vi "Write Image Header.vi"(8 "error in (no error)":errorcluster, 11 "CCDCamera in":refnum<class "CCDCamera.lvclass">) -> (0 "error out":errorcluster, 3 "CCDCamera out":refnum<class "CCDCamera.lvclass">)   [LabVIEW 2018, in "CCDCamera.lvclass"]
uses:
  CCDCamera.lvclass
  <userlib>/gfitsio/gfitsio.lvlib
  <userlib>/gfitsio/gfitsio-write-key-string.vi
panel:
  in  "Header Contents":T1={"FILENAME"=["FILENAME", "example.fits", "File name at acquisition"], "OBSERVER"=["OBSERVER", "Denis", "Name of the observer"], "PROGRID"=["PROGRID", "2018A-001", "Program ID"], "OBJECT"=["OBJECT", "UNDEFINED", "Object name"], "NIGHTDIR"=["NIGHTDIR", "DIR", "Night directory name "], "CHANNEL"=["CHANNEL", "RED", "Instrument channel"], "INSTRUME"=["INSTRUME", "ECHARPE", "Instrument"], "NEXPSEQ"=["NEXPSEQ", "1", "Total number of exposures in sequence"], "SEQINDEX"=["SEQINDEX", "1", "Exposure index in the sequence"], "OBSTYPE"=["OBSTYPE", "BIAS", "Image type: OBJECT, BIAS, FLAT, ARC, DARK"], "READOUT"=["READOUT", "Normal", "Read out rate"], "SHUTTER"=["SHUTTER", "CLOSED", "Shutter Mode (OPEN, CLOSED, or AUTO) "], "OPENSHT"=["OPENSHT", "50", "Time to open the shutter (ms) "], "CLOSESHT"=["CLOSESHT", "50", "Time to close the shutter (ms)"], "EM GAIN"=["EMGAIN", "2", "Electron Multiplying gain"], "EMMODE "=["EMMODE", "Electron Multiplying", "Electron Multiplying Mode"], "EXPTIME"=["EXPTIME", "1", "Exposure time (s)"], "PREAMP GAIN"=["PREAMP", "3.38", "Pre-amplifier gain"], "VSHIFT"=["VSHIFT", "4.33", "Vertical Shift Spedd (usec)"], "ACQMODE"=["ACQMODE", "SINGLE", "Acquisition Mode"], "TRIGGER"=["TRIGGER", "internal", "Trigger Mode"], "READMODE"=["READMODE", "Single", "Read Mode"], "SHUTTTL"=["SHUTTTL", "TTL LOW", "Shutter TTL"], "HBIN"=["HBIN", "1", "Horizontal Binning"], "INITLINE"=["INITLINE", "1", "Initial Line Multiplying gain"], "INITCOL"=["INITCOL", "1 ", "Initial Column"], "FINALLIN"=["FINALLIN", "1024", "Final Line"], "VBIN"=["VBIN", "1", "Vertical Binning"], "FINALCOL"=["FINALCOL", "1024", "Final Column"]}
  out "Camera Setup":T2={"Image Name"="Image", "Image Path"="C:\\Users\\Cliente\\Desktop\\SPARC4_AC\\Imagens\\", "# Images"="", "Exposure Time"="", "Pre-amp gain"="", "Readout Rate"="", "Vertical Shift Speed"="", "Acquisition Mode"="", "Trigger"="", "Read Mode"="", "EM Mode"="", "EM Gain"="", "Shutter Mode"="", "Shutter TTL"="", "Time to open shutter"="", "Time to close shutter"="", "Vertical Binning"="", "Horizontal Binning"="", "Initial Line"="", "Initial Cloumn"="", "Final Line"="", "Final Column"="", "#img in sequence"=""}
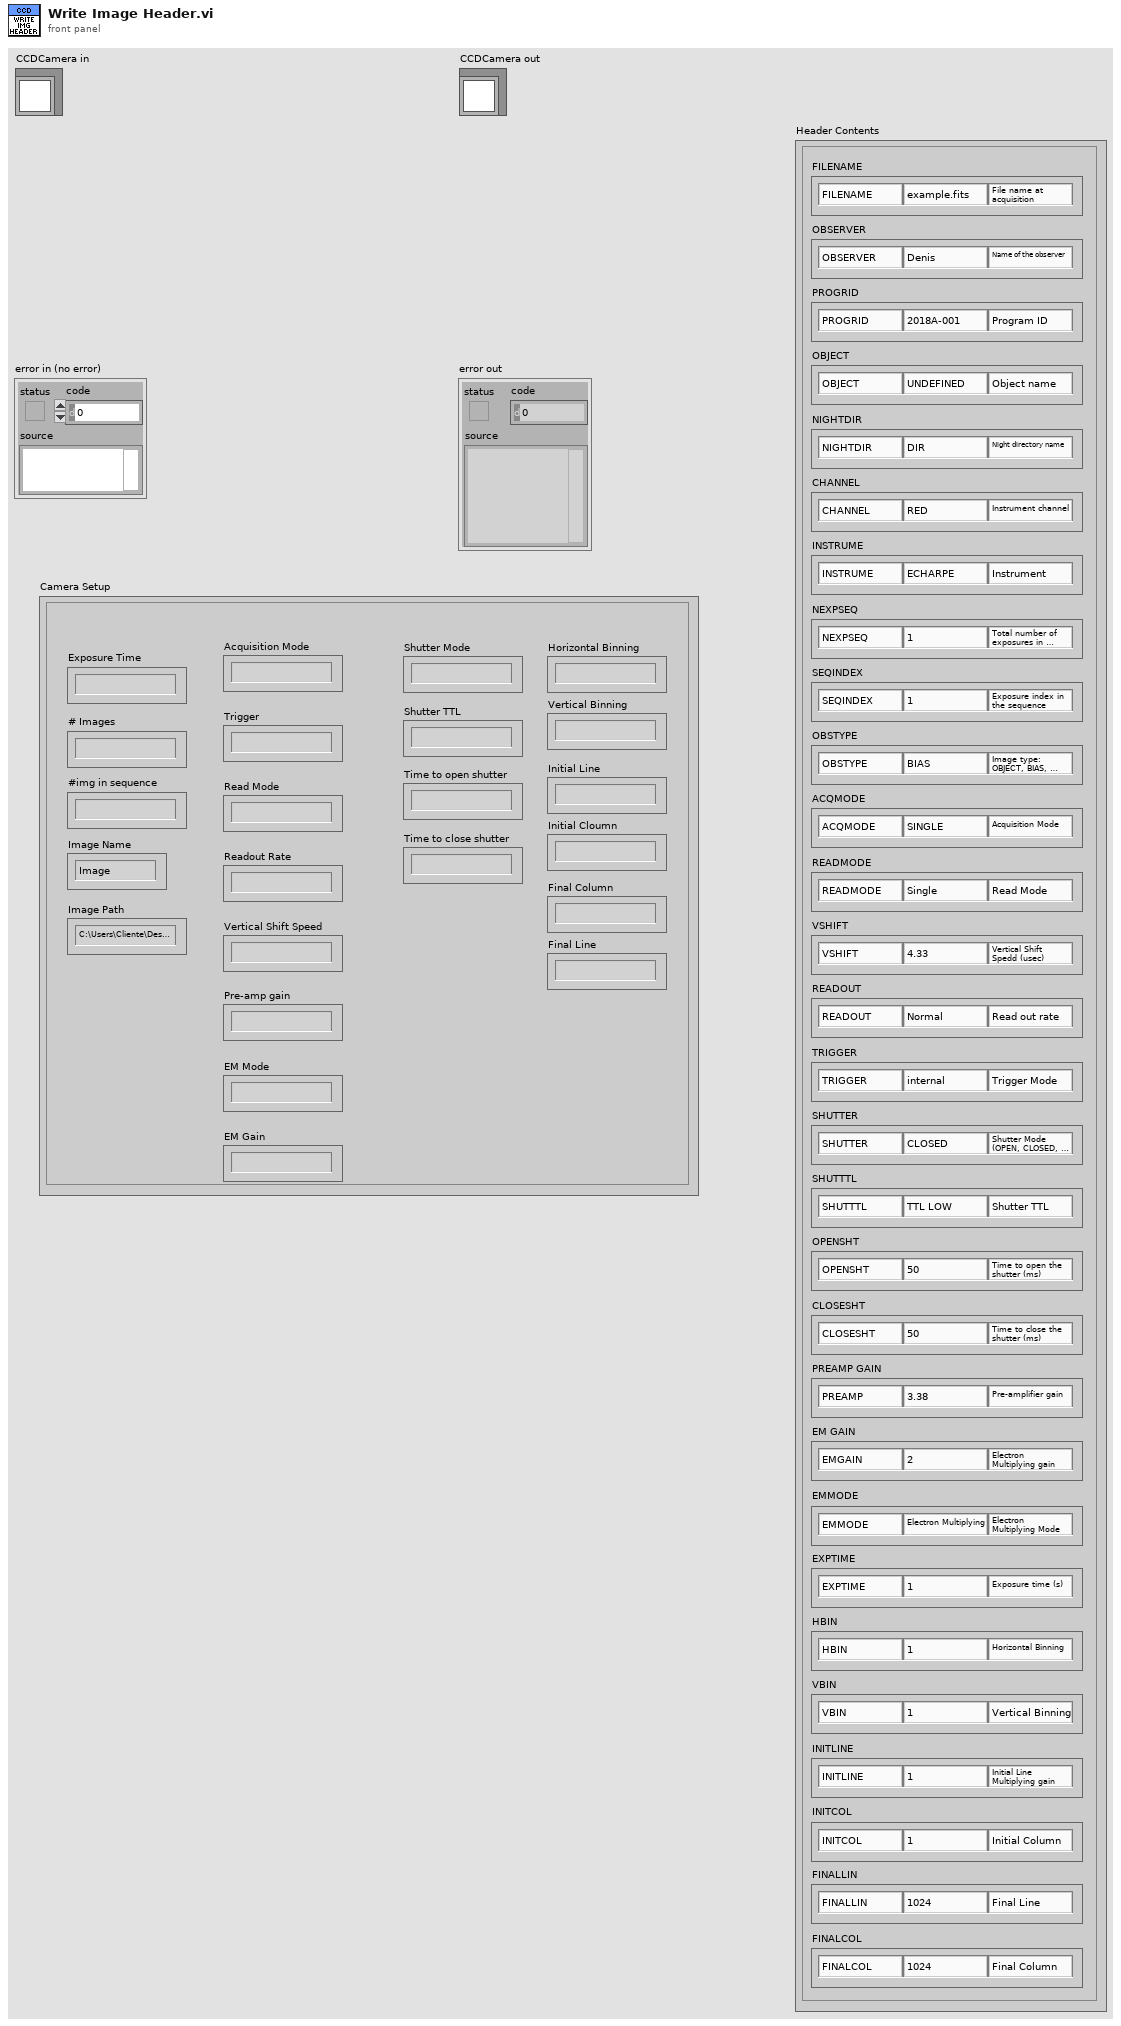
[diagram p1: front panel]
types:
  T1 = cluster{"FILENAME":string[], "OBSERVER":string[], "PROGRID":string[], "OBJECT":string[], "NIGHTDIR":string[], "CHANNEL":string[], "INSTRUME":string[], "NEXPSEQ":string[], "SEQINDEX":string[], "OBSTYPE":string[], "READOUT":string[], "SHUTTER":string[], "OPENSHT":string[], "CLOSESHT":string[], "EM GAIN":string[], "EMMODE ":string[], "EXPTIME":string[], "PREAMP GAIN":string[], "VSHIFT":string[], "ACQMODE":string[], "TRIGGER":string[], "READMODE":string[], "SHUTTTL":string[], "HBIN":string[], "INITLINE":string[], "INITCOL":string[], "FINALLIN":string[], "VBIN":string[], "FINALCOL":string[]}
  T2 = cluster{"Image Name":string, "Image Path":string, "# Images":string, "Exposure Time":string, "Pre-amp gain":string, "Readout Rate":string, "Vertical Shift Speed":string, "Acquisition Mode":string, "Trigger":string, "Read Mode":string, "EM Mode":string, "EM Gain":string, "Shutter Mode":string, "Shutter TTL":string, "Time to open shutter":string, "Time to close shutter":string, "Vertical Binning":string, "Horizontal Binning":string, "Initial Line":string, "Initial Cloumn":string, "Final Line":string, "Final Column":string, "#img in sequence":string}
  T3 = cluster{"Image Name":string, "Image Path":string, "# Images":u32, "Exposure Time":dbl, "Pre-amp gain":u8, "Readout Rate":u8, "Vertical Shift Speed":u8, "Acquisition Mode":u8, "Trigger":u8, "Read Mode":u8, "EM Mode":u8, "EM Gain":u16, "Shutter Mode":u8, "Shutter TTL":u8, "Time to open shutter":u16, "Time to close shutter":u16, "Vertical Binning":u16, "Horizontal Binning":u16, "Initial Line":u16, "Initial Column":u16, "Final Line":u16, "Final Column":u16, "Image Name (TEMP)":string, "#img in sequence":u32, "Kinetic Series Length":u32, "Number of Accumulations":u32, "Kinetic Cycle Time":u32, "Frame Transfer":bool, "Vertical Clock Amplitude":u8}
  T4 = enum16{"open", "open or create", "create or replace", "create", "open (read only)"}
  T5 = typedef "gfitsio.lvlib/gfitsio-refnum.ctl" = refnum<k1>
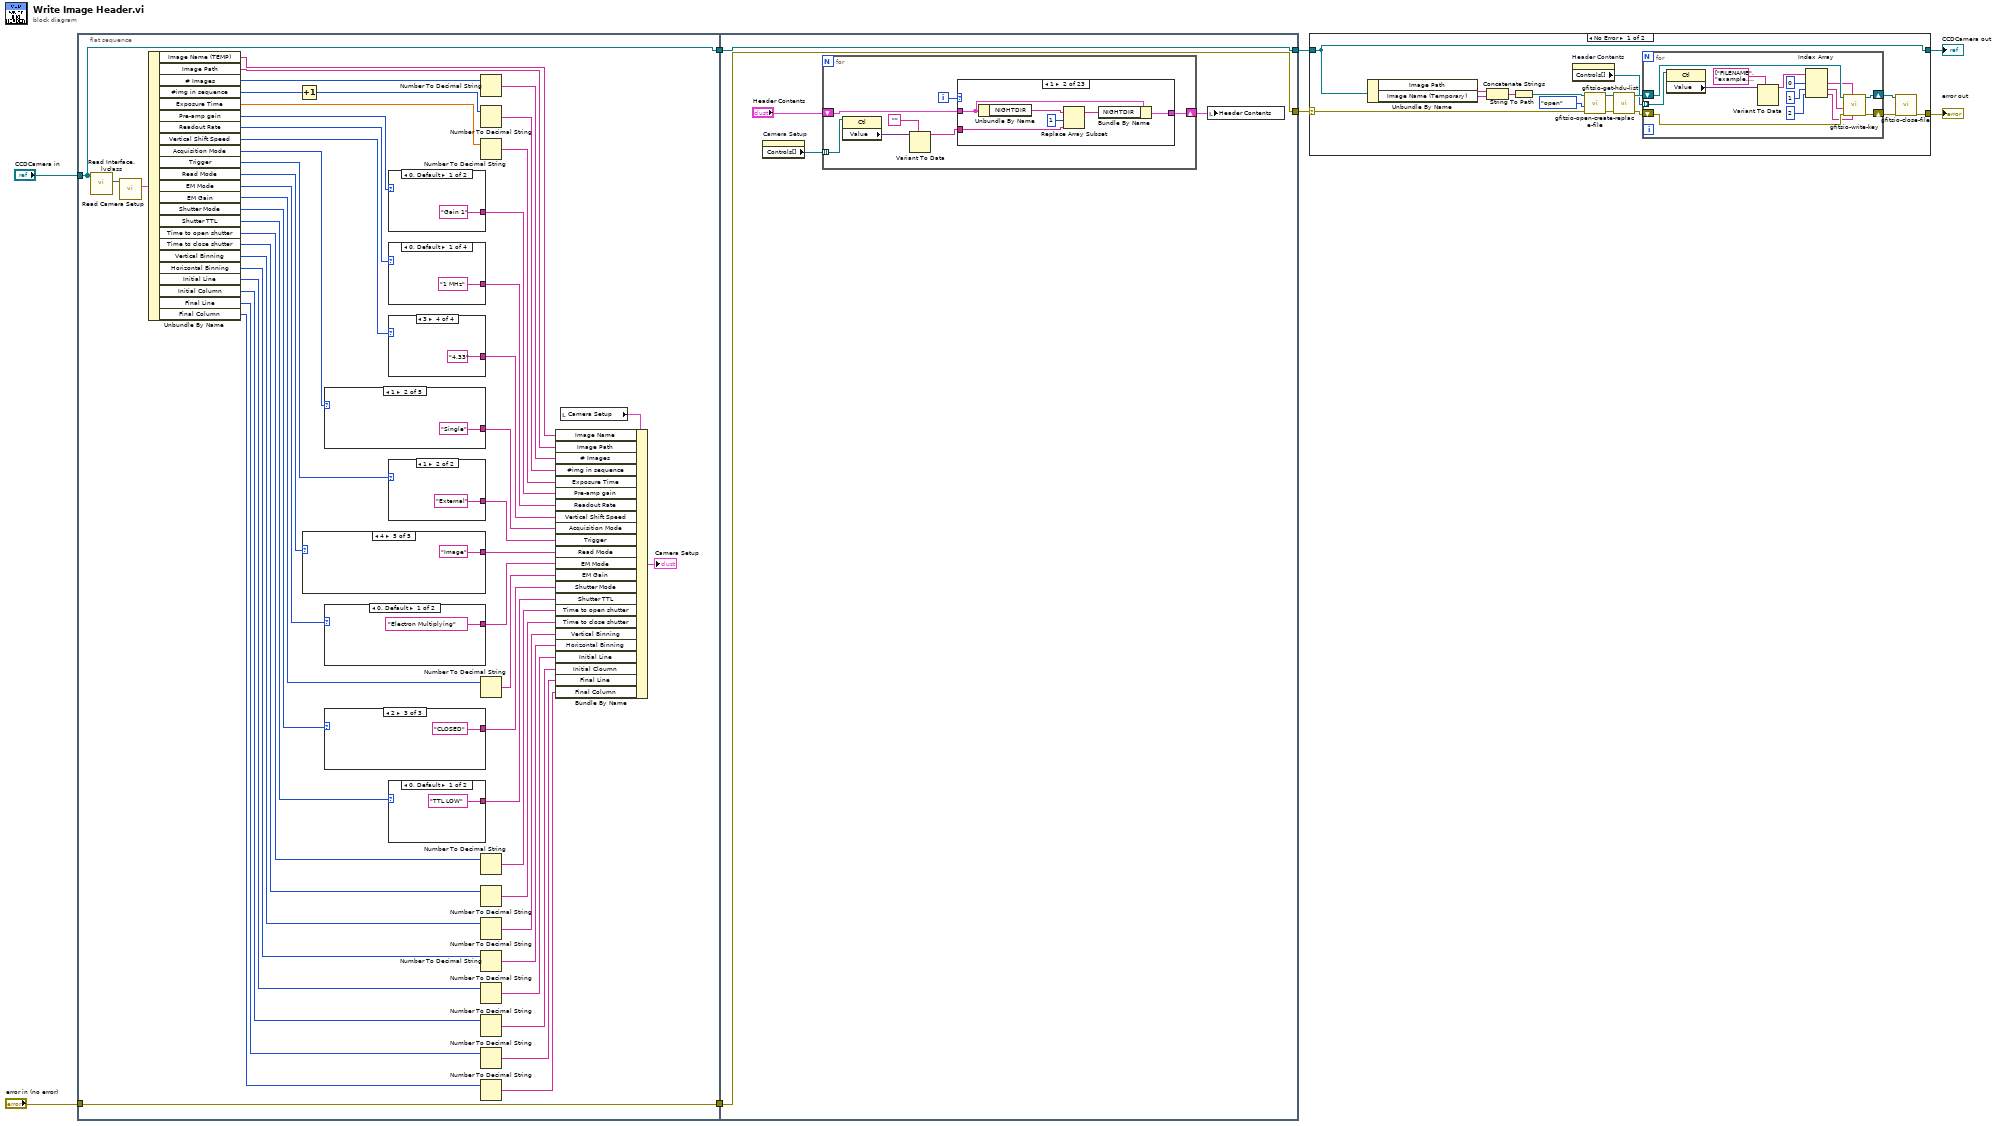
[diagram p0: block diagram]
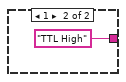
[diagram p2: hidden frame]
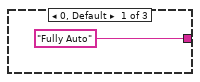
[diagram p3: hidden frame]
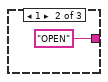
[diagram p4: hidden frame]
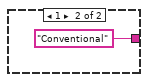
[diagram p5: hidden frame]
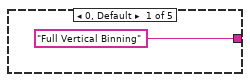
[diagram p6: hidden frame]
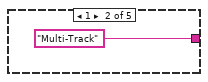
[diagram p7: hidden frame]
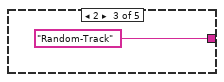
[diagram p8: hidden frame]
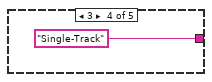
[diagram p9: hidden frame]
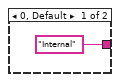
[diagram p10: hidden frame]
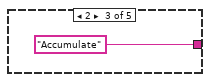
[diagram p12: hidden frame]
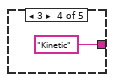
[diagram p13: hidden frame]
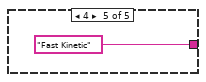
[diagram p14: hidden frame]
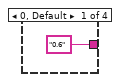
[diagram p15: hidden frame]
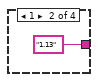
[diagram p16: hidden frame]
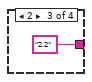
[diagram p17: hidden frame]
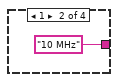
[diagram p18: hidden frame]
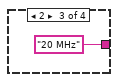
[diagram p19: hidden frame]
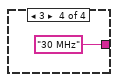
[diagram p20: hidden frame]
diagram:
  n1 = flat-sequence {
    tunnel: "CCDCamera in" -> [w13]
    tunnel: [w13] -> w5
    tunnel: [w12] -> w4
    tunnel: "error in (no error)" -> [w12]
    tunnel: w5 -> [w90]
    tunnel: w4 -> [w89]
    tunnel: [w90] -> w2
    tunnel: [w89] -> w1
    frame #0 {
      n2 = call-dynamic "Read Interface.lvclass.vi"("CCDCamera in"=w13) -> ("Interface.lvclass"=w14:refnum<class "Interface.lvclass">)  [unwired: 8 in, 2 out]
      n3 = call "Read Camera Setup.vi"("Interface in"=w14) -> ("Camera Setup"=w59:T3)  [unwired: 8 in, 2 out]
      n4 = Unbundle By Name(w59) -> ("Image Name (TEMP)"=w15:string, "Image Path"=w36:string, "# Images"=w58:u32, "#img in sequence"=w9:u32, "Exposure Time"=w57:dbl, "Pre-amp gain"=w56:u8, "Readout Rate"=w55:u8, "Vertical Shift Speed"=w54:u8, "Acquisition Mode"=w53:u8, "Trigger"=w52:u8, "Read Mode"=w51:u8, "EM Mode"=w50:u8, "EM Gain"=w49:u16, "Shutter Mode"=w48:u8, "Shutter TTL"=w47:u8, "Time to open shutter"=w46:u16, "Time to close shutter"=w45:u16, "Vertical Binning"=w43:u16, "Horizontal Binning"=w44:u16, "Initial Line"=w42:u16, "Initial Column"=w41:u16, "Final Line"=w40:u16, "Final Column"=w39:u16)
      n5 = Increment(x=w9) -> (x+1=w10:u32)
      n6 = case shown="4" w51 {
        tunnel: ["Full Vertical Binning" ("units") "Multi-Track" ("units") "Random-Track" ("units") "Single-Track" ("units") "Image" ("units")] -> w29
        frame 0, Default {
        }
        frame 1 {
        }
        frame 2 {
        }
        frame 3 {
        }
        frame 4 {
        }
      }
      n7 = case shown="1" w53 {
        tunnel: [_ "Single" ("units") "Accumulate" ("units") "Kinetic" ("units") "Fast Kinetic" ("units")] -> w31
        frame 0, Default {
        }
        frame 1 {
        }
        frame 2 {
        }
        frame 3 {
        }
        frame 4 {
        }
      }
      n8 = case shown="0, Default" w50 {
        tunnel: ["Electron Multiplying" ("units") "Conventional" ("units")] -> w28
        frame 0, Default {
        }
        frame 1 {
        }
      }
      n9 = case shown="2" w48 {
        tunnel: ["Fully Auto" ("units") "OPEN" ("units") "CLOSED" ("units")] -> w26
        frame 0, Default {
        }
        frame 1 {
        }
        frame 2 {
        }
      }
      n10 = case shown="0, Default" w56 {
        tunnel: ["Gain 1" ("units") "Gain 2" ("units")] -> w24
        frame 0, Default {
        }
        frame 1 {
        }
      }
      n11 = case shown="0, Default" w55 {
        tunnel: ["1 MHz" ("units") "10 MHz" ("units") "20 MHz" ("units") "30 MHz" ("units")] -> w33
        frame 0, Default {
        }
        frame 1 {
        }
        frame 2 {
        }
        frame 3 {
        }
      }
      n12 = case shown="3" w54 {
        tunnel: ["0.6" ("units") "1.13" ("units") "2.2" ("units") "4.33" ("units")] -> w32
        frame 0, Default {
        }
        frame 1 {
        }
        frame 2 {
        }
        frame 3 {
        }
      }
      n13 = case shown="1" w52 {
        tunnel: ["Internal" ("units") "External" ("units")] -> w30
        frame 0, Default {
        }
        frame 1 {
        }
      }
      n14 = case shown="0, Default" w47 {
        tunnel: ["TTL LOW" ("units") "TTL High" ("units")] -> w25
        frame 0, Default {
        }
        frame 1 {
        }
      }
      n15 = Number To Decimal String(number=w58) -> (decimal integer string=w35:string)  [unwired: 1 in]
      n16 = Number To Decimal String(number=w10) -> (decimal integer string=w11:string)  [unwired: 1 in]
      n17 = Number To Decimal String(number=w57) -> (decimal integer string=w34:string)  [unwired: 1 in]
      n18 = Number To Decimal String(number=w49) -> (decimal integer string=w27:string)  [unwired: 1 in]
      n19 = Number To Decimal String(number=w46) -> (decimal integer string=w23:string)  [unwired: 1 in]
      n20 = Number To Decimal String(number=w45) -> (decimal integer string=w22:string)  [unwired: 1 in]
      n21 = Number To Decimal String(number=w43) -> (decimal integer string=w21:string)  [unwired: 1 in]
      n22 = Number To Decimal String(number=w44) -> (decimal integer string=w20:string)  [unwired: 1 in]
      n23 = Number To Decimal String(number=w42) -> (decimal integer string=w19:string)  [unwired: 1 in]
      n24 = Number To Decimal String(number=w41) -> (decimal integer string=w18:string)  [unwired: 1 in]
      n25 = Number To Decimal String(number=w40) -> (decimal integer string=w17:string)  [unwired: 1 in]
      n26 = Number To Decimal String(number=w39) -> (decimal integer string=w16:string)  [unwired: 1 in]
      n27 = local read "Camera Setup"() -> (w37:T2)
      n28 = Bundle By Name(cluster=w37, "Image Name"=w15, "Image Path"=w36, "# Images"=w35, "#img in sequence"=w11, "Exposure Time"=w34, "Pre-amp gain"=w24, "Readout Rate"=w33, "Vertical Shift Speed"=w32, "Acquisition Mode"=w31, "Trigger"=w30, "Read Mode"=w29, "EM Mode"=w28, "EM Gain"=w27, "Shutter Mode"=w26, "Shutter TTL"=w25, "Time to open shutter"=w23, "Time to close shutter"=w22, "Vertical Binning"=w21, "Horizontal Binning"=w20, "Initial Line"=w19, "Initial Cloumn"=w18, "Final Line"=w17, "Final Column"=w16) -> (→"Camera Setup":T2)
    }
    frame #1 {
      n29 = property on="Camera Setup" class="Clust (strict)"() -> ("Controls[]"=w91:refnum<vi>[])  [unwired: 2 in, 2 out]
      n30 = for {
        tunnel: w91 -> [w98] mode=indexing
        shift-right: [w93] -> w88
        shift-left: "Header Contents" -> [w94]
        i -> [w99]
        n31 = property class="Ctl"(reference=w98) -> ("Value"=w96:variant)  [unwired: 1 in, 2 out]
        n32 = Variant To Data(type="", Variant=w96) -> (data=w95:string)  [unwired: 1 in, 1 out]
        n33 = case shown="1" w99 {
          tunnel: w95 -> [w103 w109 w115 w121 w127 w133 w139 w145 w151 w157 w163 w169 w175 w181 w187 w193 w199 w205 w211 w217 w223 w229 w235]
          tunnel: w94 -> [w100 w106 w112 w118 w126 w132 w138 w144 w150 w156 w162 w168 w174 w180 w186 w192 w198 w204 w210 w216 w222 w228 w234]
          tunnel: [w102 w108 w113 w120 w124 w130 w136 w142 w148 w154 w160 w166 w172 w178 w184 w190 w196 w202 w208 w214 w220 w226 w232] -> w93
          frame 0, Default {
            n34 = Unbundle By Name(w100) -> ("FILENAME"=w104:string[])
            n35 = Replace Array Subset(array=w104, new element=w103, index=1) -> (w101:string[])
            n36 = Bundle By Name(cluster=w100, "FILENAME"=w101) -> (w102:T1)
          }
          frame 1 {
            n37 = Unbundle By Name(w106) -> ("NIGHTDIR"=w110:string[])
            n38 = Replace Array Subset(array=w110, new element=w109, index=1) -> (w107:string[])
            n39 = Bundle By Name(cluster=w106, "NIGHTDIR"=w107) -> (w108:T1)
          }
          frame 2 {
            n40 = Unbundle By Name(w112) -> ("NEXPSEQ"=w116:string[])
            n41 = Replace Array Subset(array=w116, new element=w115, index=1) -> (w114:string[])
            n42 = Bundle By Name(cluster=w112, "NEXPSEQ"=w114) -> (w113:T1)
          }
          frame 3 {
            n43 = Unbundle By Name(w118) -> ("EXPTIME"=w122:string[])
            n44 = Replace Array Subset(array=w122, new element=w121, index=1) -> (w119:string[])
            n45 = Bundle By Name(cluster=w118, "EXPTIME"=w119) -> (w120:T1)
          }
          frame 4 {
            n46 = Unbundle By Name(w126) -> ("PREAMP GAIN"=w128:string[])
            n47 = Replace Array Subset(array=w128, new element=w127, index=1) -> (w125:string[])
            n48 = Bundle By Name(cluster=w126, "PREAMP GAIN"=w125) -> (w124:T1)
          }
          frame 5 {
            n49 = Unbundle By Name(w132) -> ("READOUT"=w134:string[])
            n50 = Replace Array Subset(array=w134, new element=w133, index=1) -> (w131:string[])
            n51 = Bundle By Name(cluster=w132, "READOUT"=w131) -> (w130:T1)
          }
          frame 6 {
            n52 = Unbundle By Name(w138) -> ("VSHIFT"=w140:string[])
            n53 = Replace Array Subset(array=w140, new element=w139, index=1) -> (w137:string[])
            n54 = Bundle By Name(cluster=w138, "VSHIFT"=w137) -> (w136:T1)
          }
          frame 7 {
            n55 = Unbundle By Name(w144) -> ("ACQMODE"=w146:string[])
            n56 = Replace Array Subset(array=w146, new element=w145, index=1) -> (w143:string[])
            n57 = Bundle By Name(cluster=w144, "ACQMODE"=w143) -> (w142:T1)
          }
          frame 8 {
            n58 = Unbundle By Name(w150) -> ("TRIGGER"=w152:string[])
            n59 = Replace Array Subset(array=w152, new element=w151, index=1) -> (w149:string[])
            n60 = Bundle By Name(cluster=w150, "TRIGGER"=w149) -> (w148:T1)
          }
          frame 9 {
            n61 = Unbundle By Name(w156) -> ("READMODE"=w158:string[])
            n62 = Replace Array Subset(array=w158, new element=w157, index=1) -> (w155:string[])
            n63 = Bundle By Name(cluster=w156, "READMODE"=w155) -> (w154:T1)
          }
          frame 10 {
            n64 = Unbundle By Name(w162) -> ("EMMODE"=w164:string[])
            n65 = Replace Array Subset(array=w164, new element=w163, index=1) -> (w161:string[])
            n66 = Bundle By Name(cluster=w162, "EMMODE"=w161) -> (w160:T1)
          }
          frame 11 {
            n67 = Unbundle By Name(w168) -> ("EM GAIN"=w170:string[])
            n68 = Replace Array Subset(array=w170, new element=w169, index=1) -> (w167:string[])
            n69 = Bundle By Name(cluster=w168, "EM GAIN"=w167) -> (w166:T1)
          }
          frame 12 {
            n70 = Unbundle By Name(w174) -> ("SHUTTER"=w176:string[])
            n71 = Replace Array Subset(array=w176, new element=w175, index=1) -> (w173:string[])
            n72 = Bundle By Name(cluster=w174, "SHUTTER"=w173) -> (w172:T1)
          }
          frame 13 {
            n73 = Unbundle By Name(w180) -> ("SHUTTTL"=w182:string[])
            n74 = Replace Array Subset(array=w182, new element=w181, index=1) -> (w179:string[])
            n75 = Bundle By Name(cluster=w180, "SHUTTTL"=w179) -> (w178:T1)
          }
          frame 14 {
            n76 = Unbundle By Name(w186) -> ("OPENSHT"=w188:string[])
            n77 = Replace Array Subset(array=w188, new element=w187, index=1) -> (w185:string[])
            n78 = Bundle By Name(cluster=w186, "OPENSHT"=w185) -> (w184:T1)
          }
          frame 15 {
            n79 = Unbundle By Name(w192) -> ("CLOSESHT"=w194:string[])
            n80 = Replace Array Subset(array=w194, new element=w193, index=1) -> (w191:string[])
            n81 = Bundle By Name(cluster=w192, "CLOSESHT"=w191) -> (w190:T1)
          }
          frame 16 {
            n82 = Unbundle By Name(w198) -> ("VBIN"=w200:string[])
            n83 = Replace Array Subset(array=w200, new element=w199, index=1) -> (w197:string[])
            n84 = Bundle By Name(cluster=w198, "VBIN"=w197) -> (w196:T1)
          }
          frame 17 {
            n85 = Unbundle By Name(w204) -> ("HBIN"=w206:string[])
            n86 = Replace Array Subset(array=w206, new element=w205, index=1) -> (w203:string[])
            n87 = Bundle By Name(cluster=w204, "HBIN"=w203) -> (w202:T1)
          }
          frame 18 {
            n88 = Unbundle By Name(w210) -> ("INITLINE"=w212:string[])
            n89 = Replace Array Subset(array=w212, new element=w211, index=1) -> (w209:string[])
            n90 = Bundle By Name(cluster=w210, "INITLINE"=w209) -> (w208:T1)
          }
          frame 19 {
            n91 = Unbundle By Name(w216) -> ("INITCOL"=w218:string[])
            n92 = Replace Array Subset(array=w218, new element=w217, index=1) -> (w215:string[])
            n93 = Bundle By Name(cluster=w216, "INITCOL"=w215) -> (w214:T1)
          }
          frame 20 {
            n94 = Unbundle By Name(w222) -> ("FINALLIN"=w224:string[])
            n95 = Replace Array Subset(array=w224, new element=w223, index=1) -> (w221:string[])
            n96 = Bundle By Name(cluster=w222, "FINALLIN"=w221) -> (w220:T1)
          }
          frame 21 {
            n97 = Unbundle By Name(w228) -> ("FINALCOL"=w230:string[])
            n98 = Replace Array Subset(array=w230, new element=w229, index=1) -> (w227:string[])
            n99 = Bundle By Name(cluster=w228, "FINALCOL"=w227) -> (w226:T1)
          }
          frame 22 {
            n100 = Unbundle By Name(w234) -> ("SEQINDEX"=w236:string[])
            n101 = Replace Array Subset(array=w236, new element=w235, index=1) -> (w233:string[])
            n102 = Bundle By Name(cluster=w234, "SEQINDEX"=w233) -> (w232:T1)
          }
        }
      }
      n103 = local write "Header Contents"(w88) -> ()
    }
  }
  n104 = case shown="No Error" w1 {
    selector: w1 -> [w238 w268]
    tunnel: [w243 w268] -> w8
    tunnel: [w239 w267] -> w7
    tunnel: w2 -> [w239 w267]
    frame No Error {
      n105 = Unbundle By Name(w239) -> ("Image Path"=w252:string, "Image Name (Temporary)"=w240:string)
      n106 = Concatenate Strings(w252, w240) -> (w251:string)
      n107 = String To Path(string=w251) -> (path=w250:path)
      n108 = property on="Header Contents" class="Clust (strict)"() -> ("Controls[]"=w241:refnum<vi>[])  [unwired: 2 in, 2 out]
      n109 = call <userlib>:"gfitsio-open-create-replace-file.vi"("error in (no error)"=w238, "function (open)"=T4."open", "file path (dialog if empty)"=w250) -> ("error out"=w249:errorcluster, "gfits refnum"=w248:T5)  [unwired: 6 in, 1 out]
      n110 = call <userlib>:"gfitsio-get-hdu-list.vi"("error in (no error)"=w249, "gfits refnum"=w248) -> ("error out"=w246:errorcluster, "dup gfits refnum"=w247:T5)  [unwired: 6 in, 2 out]
      n111 = for {
        shift-right: [w266] -> w244
        shift-left: w247 -> [w264]
        shift-right: [w265] -> w245
        shift-left: w246 -> [w263]
        tunnel: w241 -> [w260] mode=indexing
        n112 = property class="Ctl"(reference=w260) -> ("Value"=w262:variant)  [unwired: 1 in, 2 out]
        n113 = Variant To Data(type=string[] ["FILENAME", "example.fits", "File name at acquisition"] ("FILENAME"), Variant=w262) -> (data=w259:string[])  [unwired: 1 in, 1 out]
        n114 = Index Array(array=w259, index #1=0, index #2=1, index #3=2) -> (element #1=w255:string, element #2=w254:string, element #3=w253:string)
        n115 = call-poly <userlib>:"gfitsio-write-key.vi"("comment"=w253, "keyname"=w255, "error in (no error)"=w263, "value"=w254, "gfits refnum"=w264) -> ("error out"=w265:errorcluster, "dup gfits refnum"=w266:T5)  [unwired: 5 in]
      }
      n116 = call <userlib>:"gfitsio-close-file.vi"("error in (no error)"=w245, "gfits refnum"=w244) -> ("error out"=w243:errorcluster)  [unwired: 8 in, 1 out]
    }
    frame Error {
    }
  }
  "error out" <- w8
  "CCDCamera out" <- w7
